vi "Configure Frequency Offset.vi"(0 "VISA resource name":refnum<visa-resource-name>, 1 "Multiplier (1)":dbl=1.0, 2 "Divisor (1)":dbl=1.0, 5 "Channel (1)":i32=1, 7 "Offset Frequency (0 Hz)":dbl, 9 "CW Override State (F: Disable)":bool, 11 "error in (no error)":errorcluster, 12 "Enable Offset State (F: Disable)":bool) -> (4 "VISA resource name out":refnum<visa-resource-name>, 15 "error out":errorcluster)   [LabVIEW 2018, in "Keysight PNA Series.lvlib"]
doc: "Configures frequency offset."
uses:
  Keysight PNA Series.lvlib
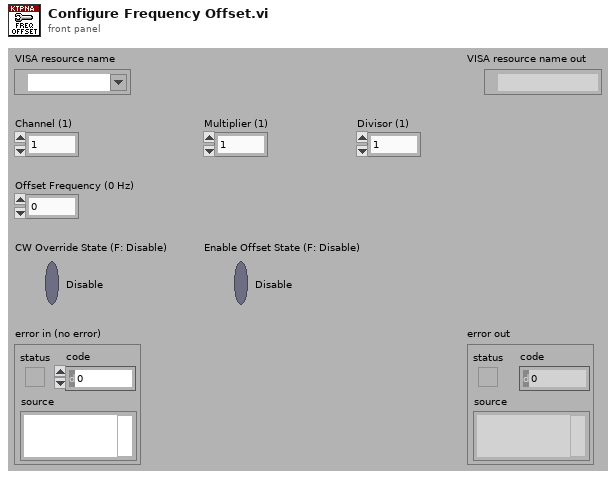
[diagram p1: front panel]
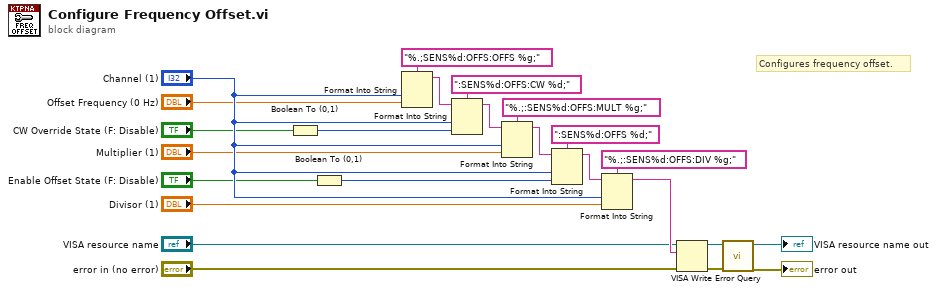
[diagram p0: block diagram]
diagram:
  # "Configures frequency offset."
  n1 = Boolean To (0,1)(Boolean="CW Override State (F: Disable)") -> (0, 1=w3:i16)
  n2 = Boolean To (0,1)(Boolean="Enable Offset State (F: Disable)") -> (0, 1=w1:i16)
  n3 = Format Into String(format string="%.;SENS%d:OFFS:OFFS %g;", "Channel (1)", "Offset Frequency (0 Hz)") -> (resulting string=w21:string)  [unwired: 2 in, 1 out]
  n4 = Format Into String(format string=":SENS%d:OFFS:CW %d;", initial string=w21, "Channel (1)", w3) -> (resulting string=w19:string)  [unwired: 1 in, 1 out]
  n5 = Format Into String(format string="%.;:SENS%d:OFFS:MULT %g;", initial string=w19, "Channel (1)", "Multiplier (1)") -> (resulting string=w16:string)  [unwired: 1 in, 1 out]
  n6 = Format Into String(format string=":SENS%d:OFFS %d;", initial string=w16, "Channel (1)", w1) -> (resulting string=w14:string)  [unwired: 1 in, 1 out]
  n7 = Format Into String(format string="%.;:SENS%d:OFFS:DIV %g;", initial string=w14, "Channel (1)", "Divisor (1)") -> (resulting string=w11:string)  [unwired: 1 in, 1 out]
  n8 = VISA Write(VISA resource name="VISA resource name", write buffer=w11, error in (no error)="error in (no error)") -> (VISA resource name out=w8:refnum<visa-resource-name>, error out=w7:errorcluster)  [unwired: 1 out]
  n9 = call "Error Query.vi"("error in (no error)"=w7, "VISA resource name"=w8) -> ("error out"=→"error out":errorcluster, "VISA resource name out"=→"VISA resource name out":refnum<visa-resource-name>)  [unwired: 6 in, 2 out]
